vi "LFA_Capture.vi"(8 "error in (no error)":errorcluster, 10 "Frames":i32, 11 "LightField Automation in":refnum<class "LightField Automation.lvclass">) -> (0 "error out":errorcluster, 2 "Data":T1(array[cluster]), 3 "LightField Automation out":refnum<class "LightField Automation.lvclass">)   [LabVIEW 2018, in "LightField Automation.lvclass"]
uses:
  LightField Automation.lvclass
  LightField Automation.lvclass/LightField Automation.ctl
  C:/Users/xw9/Desktop/Turbulence program/SourceDistribution/PrincetonInstruments.LightFieldViewV3.dll
  PrincetonInstruments.LightFieldViewV3.dll
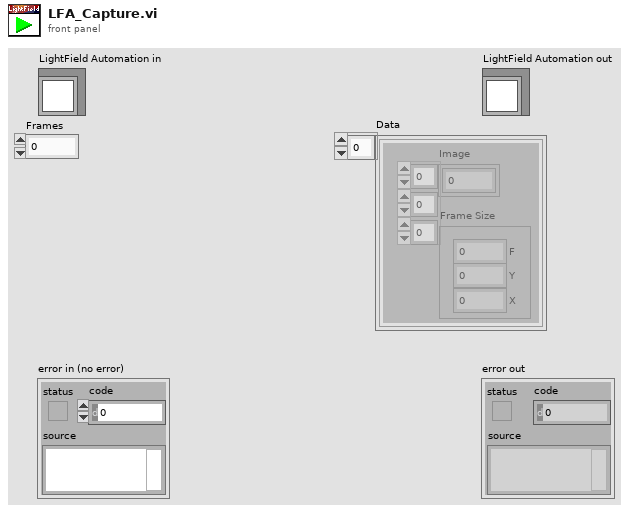
[diagram p1: front panel]
types:
  T1 = cluster{"Image":dbl[][][], "Frame Size":cluster{"F":i32, "Y":i32, "X":i32}}[]
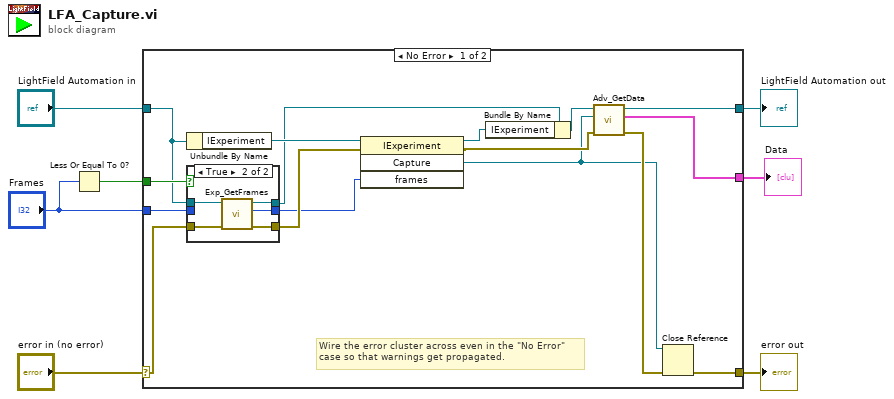
[diagram p0: block diagram]
diagram:
  n1 = Less Or Equal To 0?(x="Frames") -> (x <= 0?=w2:bool)
  n2 = case shown="No Error" "error in (no error)" {
    selector: "error in (no error)" -> [w19 w33]
    tunnel: [w9 w33] -> w6
    tunnel: [w22 w32] -> w4
    tunnel: "LightField Automation in" -> [w18 w32]
    tunnel: [w21 _] -> w3
    tunnel: w2 -> [w20 _]
    tunnel: "Frames" -> [w16 _]
    frame No Error {
      # "Wire the error cluster across even in the \"No Error\"\ncase so that warnings get propagated."
      n3 = Unbundle By Name(w18) -> ("IExperiment"=w23:refnum<k24>)
      n4 = case shown="True" w20 {
        tunnel: w19 -> [w25 w31]
        tunnel: w18 -> [w26 w30]
        tunnel: [w26 w29] -> w14
        tunnel: [w25 w28] -> w17
        tunnel: [w24 w27] -> w11
        tunnel: w16 -> [w24 _]
        frame False {
        }
        frame True {
          n5 = call "Exp_GetFrames.vi"("error in (no error)"=w31, "LightField Automation in"=w30) -> ("error out"=w28:errorcluster, "Frames"=w27:i32, "LightField Automation out"=w29:refnum<class "LightField Automation.lvclass">)  [unwired: 7 in]
        }
      }
      n6 = invoke class="IExperiment" method="Capture"(reference=w23, error in=w17, "frames"=w11) -> (reference out=w12:refnum<k24>, error out=w15:errorcluster, "Capture"=w8:refnum<k24>)  [unwired: 1 in, 1 out]
      n7 = Bundle By Name(cluster=w14, "IExperiment"=w12) -> (w13:refnum<class "LightField Automation.lvclass">)
      n8 = call "Adv_GetData.vi"("error in (no error)"=w15, "IImageDataSet"=w8, "LightField Automation in"=w13) -> ("error out"=w10:errorcluster, "Data"=w21:T1, "LightField Automation out"=w22:refnum<class "LightField Automation.lvclass">)  [unwired: 6 in]
      n9 = Close Reference(reference=w8, error in (no error)=w10) -> (error out=w9:errorcluster)
    }
    frame Error {
    }
  }
  "error out" <- w6
  "LightField Automation out" <- w4
  "Data" <- w3
